vi "Read.vi"(7 "mode":T1(ring)=enum."Buffered", 8 "error in (no error)":errorcluster, 9 "timeout (ms)":i32=500, 10 "bytes to read":i32, 11 "TCP_Streamer_Subscriber in":refnum<class "TCP_Streamer_Subscriber.lvclass">) -> (0 "error out":errorcluster, 1 "Timeout":bool, 2 "data out":string, 3 "TCP_Streamer_Subscriber out":refnum<class "TCP_Streamer_Subscriber.lvclass">)   [LabVIEW 2021, in "TCP_Streamer_Subscriber.lvclass"]
doc: "Wraps the standard TCP read with connection and error management. It is recommended to use mode buffered for streaming to avoid partial reads from the streaming sender. \n\nSee standard TCP Read for additional help."
uses:
  TCP_Streamer_Subscriber.lvclass
  TCP_Streamer_Subscriber.lvclass/TCP_Streamer_Subscriber.ctl
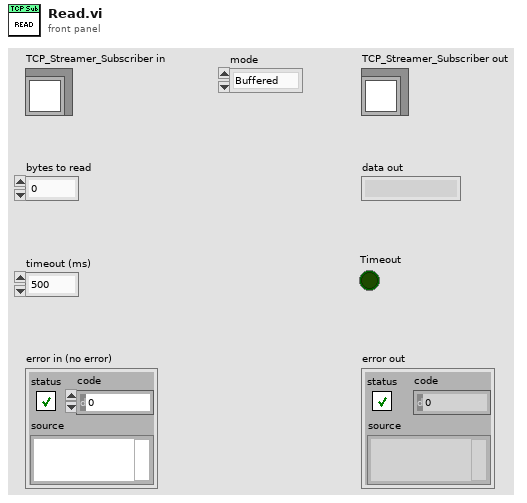
[diagram p1: front panel]
types:
  T1 = enum16{"Standard", "Buffered", "CRLF", "Immediate"}
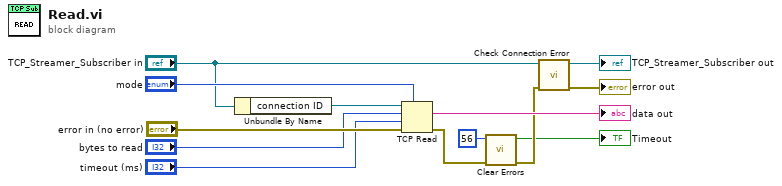
[diagram p0: block diagram]
diagram:
  n1 = Unbundle By Name("TCP_Streamer_Subscriber in") -> ("connection ID"=w12:refnum<k5>)
  n2 = TCP Read(connection ID=w12, bytes to read="bytes to read", error in (no error)="error in (no error)", 7:"mode", 9:"timeout (ms)") -> (data out=→"data out":string, error out=w4:errorcluster)  [unwired: 1 out]
  n3 = call <vilib>:"Clear Errors.vi"("error in (no error)"=w4, "specific error code to clear (0: all)"=56) -> ("error out"=w3:errorcluster, "specific error cleared?"=→"Timeout":bool)  [unwired: 4 in]
  n4 = call "Check Connection Error.vi"("error in (no error)"=w3, "TCP_Streamer_Subscriber in"="TCP_Streamer_Subscriber in") -> ("error out"=→"error out":errorcluster, "TCP_Streamer_Subscriber out"=→"TCP_Streamer_Subscriber out":refnum<class "TCP_Streamer_Subscriber.lvclass">)  [unwired: 8 in]
